vi "Thev-L to Fq.vi"(1 "L (mm)":dbl) -> (0 "Fq (Hz)":dbl)   [LabVIEW 2015]
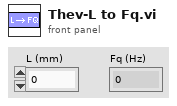
[diagram p1: front panel]
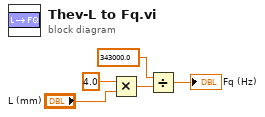
[diagram p0: block diagram]
diagram:
  n1 = Multiply(x=4.0, y="L (mm)") -> (x*y=w3:dbl)
  n2 = Divide(x=343000.0, y=w3) -> (x/y=→"Fq (Hz)":dbl)
